vi "AddVariable.vi"(6 "type":T1 items=["Boolean"=1, "SByte"=2, "Byte"=3, "Int16"=4, "UInt16"=5, "Int32"=6, "UInt32"=7, "Int64"=8, "UInt64"=9, "Float"=10, "Double"=11, "String"=12, "DateTime"=13, "ByteString"=15, "Array of Boolean"=101, "Array of SByte"=102, "Array of Byte"=103, "Array of Int16"=104, "Array of UInt16"=105, "Array of Int32"=106, "Array of UInt32"=107, "Array of Int64"=108, "Array of UInt64"=109, "Array of Float"=110, "Array of Double"=111, "Array of String"=112, "Array of DateTime"=113, "Array of ByteString"=115, "Matrix of Boolean"=201, "Matrix of SByte"=202, "Matrix of Byte"=203, "Matrix of Int16"=204, "Matrix of UInt16"=205, "Matrix of Int32"=206, "Matrix of UInt32"=207, "Matrix of Int64"=208, "Matrix of UInt64"=209, "Matrix of Float"=210, "Matrix of Double"=211, "Matrix of String "=212, "Matrix of DateTime"=213, "Matrix of ByteString"=215], 7 "variable_node":string, 8 "error in (no error)":errorcluster, 9 "variable_browse":string, 10 "variable_display":string, 11 "Server in":refnum<class "Server.lvclass">) -> (0 "error out":errorcluster, 3 "Server out":refnum<class "Server.lvclass">)   [LabVIEW 2017, in "opcua.lvlib" / "Server.lvclass"]
uses:
  Server.lvclass
  TypeDefs/Data Type.ctl
  Server.lvclass/Server.ctl
  opcua32.dll
  opcua.lvlib
panel:
  in  "ns":i32=2
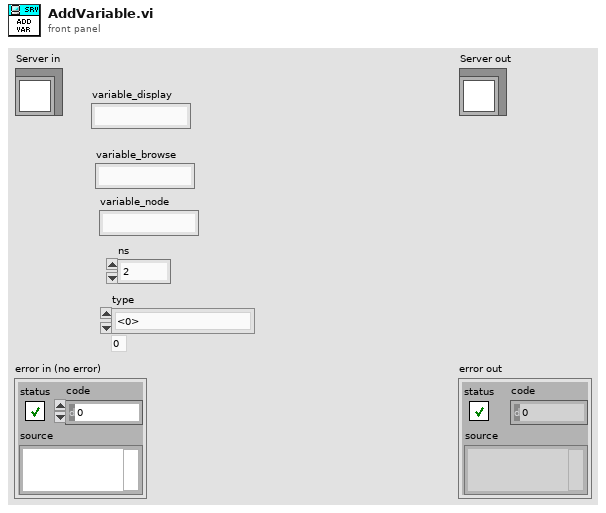
[diagram p1: front panel]
types:
  T1 = typedef "opcua.lvlib/Data Type.ctl" = u16
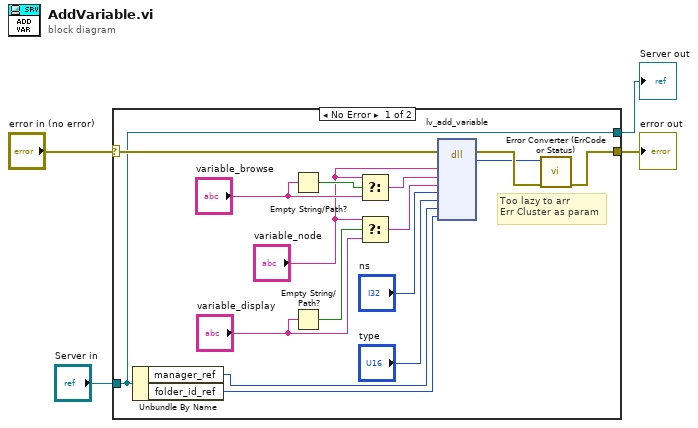
[diagram p0: block diagram]
diagram:
  n1 = case shown="No Error" "error in (no error)" {
    selector: "error in (no error)" -> [w19 w21]
    tunnel: [w6 w21] -> w3
    tunnel: [w16 w22] -> w1
    tunnel: "Server in" -> [w16 w22]
    frame No Error {
      # "Too lazy to arr\nErr Cluster as param"
      n2 = Unbundle By Name(w16) -> ("manager_ref"=w20:u64, "folder_id_ref"=w17:u64)
      n3 = Empty String/Path?(string/path="variable_browse") -> (empty?=w13:bool)
      n4 = Empty String/Path?(string/path="variable_display") -> (empty?=w14:bool)
      n5 = Select(t="variable_node", s=w13, f="variable_browse") -> (s? t:f=w11:string)
      n6 = Select(t="variable_node", s=w14, f="variable_display") -> (s? t:f=w8:string)
      n7 = dll-call lib="C:/Users/Andrey/Desktop/opcua-labview/opcua-lvlib/opcua*.dll" fn="lv_add_variable"(error in=w19, "folder_node"="variable_node", "folder_browse"=w11, "folder_display"=w8, "ns"="ns", "type"="type", "manager"=w20, "folder_id_in"=w17) -> (error out=w7:errorcluster, "return type"=w5:i32)  [unwired: 9 in, 1 out]
      n8 = call "Error Converter (ErrCode or Status).vi"("error in (no error)"=w7, "error code"=w5) -> ("error out"=w6:errorcluster)  [unwired: 9 in]
    }
    frame Error {
    }
  }
  "error out" <- w3
  "Server out" <- w1
